vi "Skew_Image2.vi"(4 "[IN] Skewed Image":T1, 5 "[IN] Share Angle":u16 max=89 step=1, 6 "[IN] Calculation mode":enum16{"Single core", "2x cores", "4x cores"}(ring), 7 "error IN":errorcluster, 8 "[IN] Y = Array rows":i32, 9 "[IN] X = Array cols":i32, 10 "[IN] Source Image U16":u16[][](array[numeric])) -> (0 "error OUT":errorcluster, 3 "[OUT] Skewed Image":T1)   [LabVIEW 2020]
uses:
  <vilib>/vision/Image Controls.llb/IMAQ Image.ctl
  <vilib>/vision/NI_Vision_Development_Module.lvlib
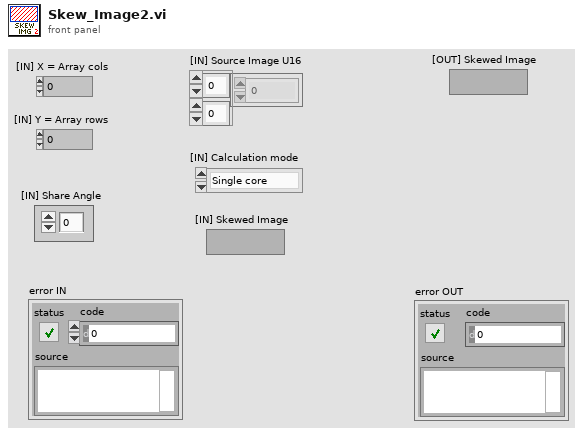
[diagram p1: front panel]
types:
  T1 = typedef "IMAQ Image.ctl" = refnum<image>
  T2 = typedef "Image Type" = u32
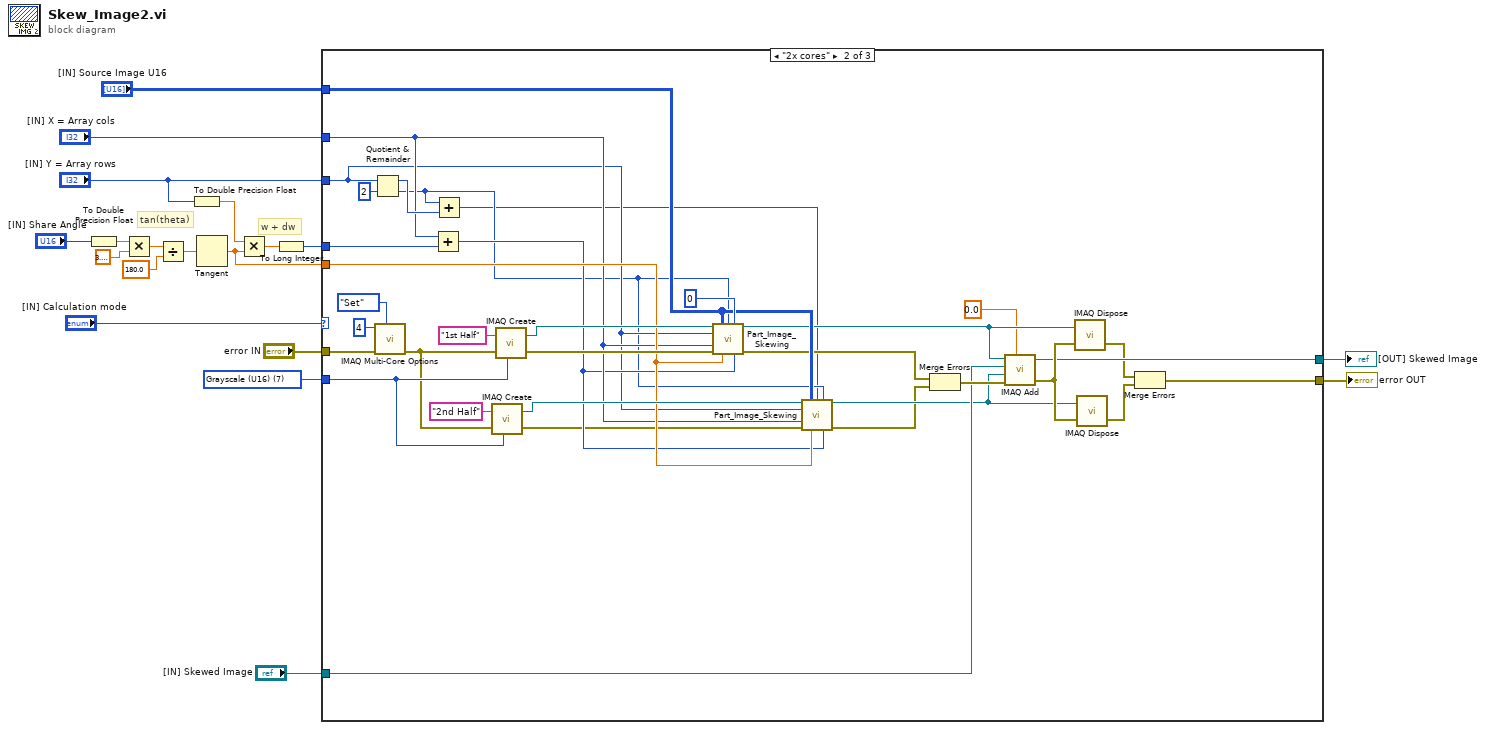
[diagram p0: block diagram]
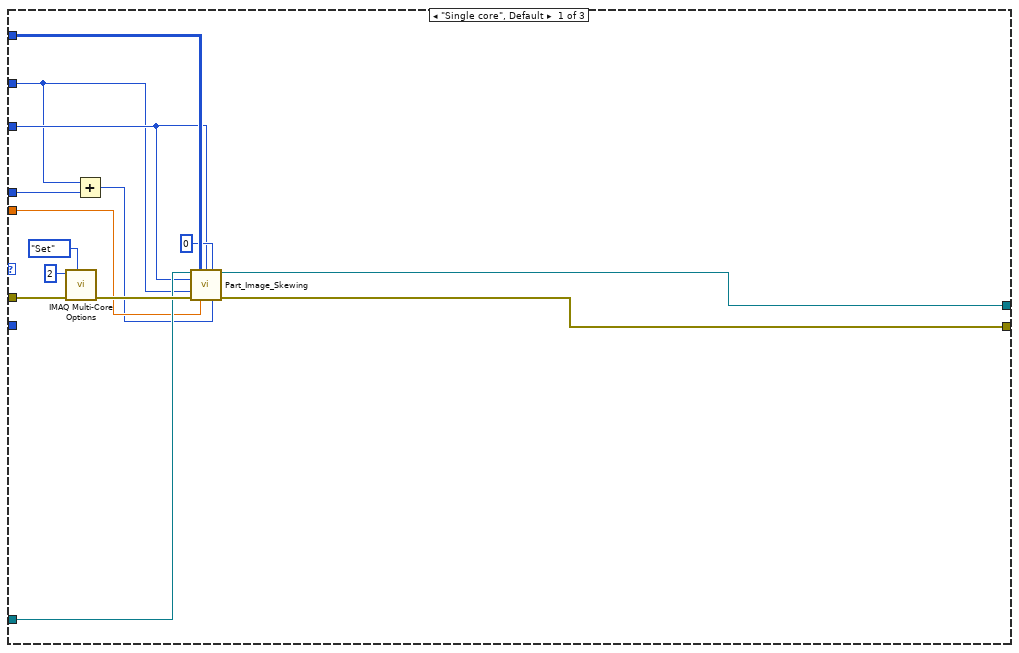
[diagram p2: hidden frame]
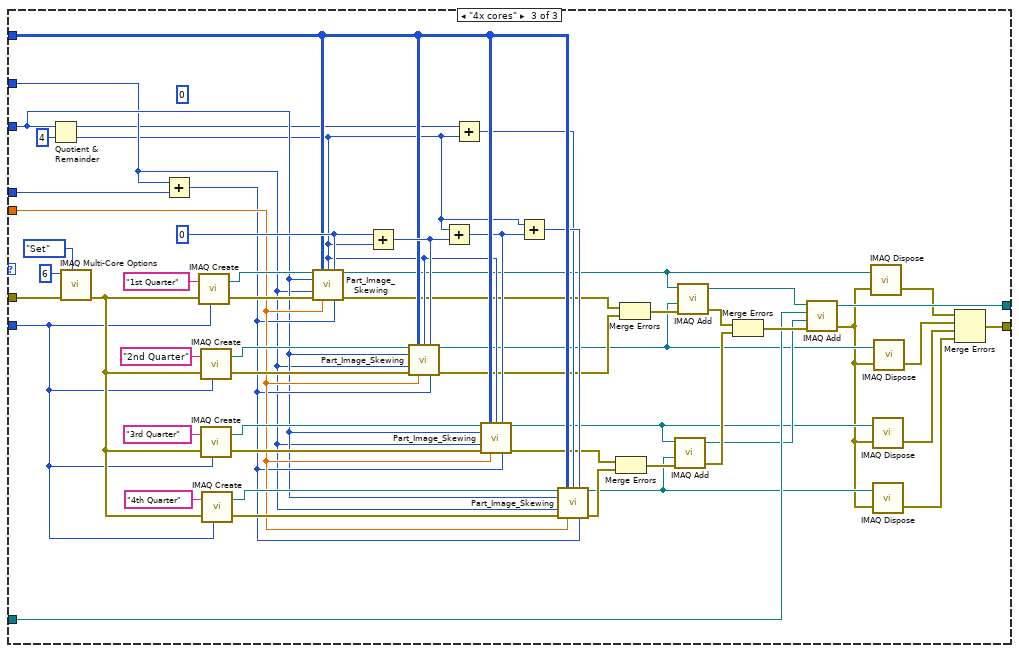
[diagram p3: hidden frame]
diagram:
  w3 = T2 7 items=["Grayscale (U8)", "Grayscale (I16)", "Grayscale (SGL)", "Complex (CSG)", "RGB (U32)", "HSL (U32)", "RGB (U64)", "Grayscale (U16)"] ("Image Type")
  # "w + dw"
  # "tan(theta)"
  n1 = To Double Precision Float(number="[IN] Share Angle") -> (double precision float=w19:dbl)
  n2 = Multiply(x=w19, y=3.141592653589793) -> (x*y=w18:dbl)
  n3 = Divide(x=w18, y=180.0) -> (x/y=w16:dbl)
  n4 = To Double Precision Float(number="[IN] Y = Array rows") -> (double precision float=w10:dbl)
  n5 = Tangent(1:w16) -> (0:w14:dbl)
  n6 = Multiply(x=w10, y=w14) -> (x*y=w13:dbl)
  n7 = To Long Integer(number=w13) -> (32bit integer=w15:i32)
  n8 = case shown="\"2x cores\"" "[IN] Calculation mode" {
    tunnel: w15 -> [w23 w66 w120]
    tunnel: w14 -> [w21 w50 w100]
    tunnel: "[IN] Source Image U16" -> [w28 w53 w96]
    tunnel: "[IN] X = Array cols" -> [w22 w49 w97]
    tunnel: "[IN] Y = Array rows" -> [w24 w39 w98]
    tunnel: "error IN" -> [w31 w59 w117]
    tunnel: [w25 w40 w72] -> w4
    tunnel: w3 -> [_ w60 w111]
    tunnel: [w26 w43 w76] -> w2
    tunnel: "[IN] Skewed Image" -> [w29 w47 w80]
    frame "Single core", Default {
      n9 = call "IMAQ Multi-Core Options"("Get/Set Number of Cores (Get)"=enum32{"Get", "Set", "Set Max Available"}."Set", "error in (no error)"=w31, "Specified Number of Cores"=u32 2) -> ("error out"=w30:errorcluster)  [unwired: 7 in, 1 out]
      n10 = Add(x=w22, y=w23) -> (x+y=w20:i32)
      n11 = call "Part_Image_Skewing.vi"("[IN] Part Image"=w29, "[IN] Source Image U16"=w28, "[IN] Rows Part"=w24, "[IN] Part shift"=0, "[IN] Rows"=w24, "[IN] Cols Initial"=w22, "error IN"=w30, "[IN] tan(theta)"=w21, "[IN] Cols"=w20) -> ("[OUT] Part Image"=w26:T1, "error OUT"=w25:errorcluster)  [unwired: 5 in]
    }
    frame "2x cores" {
      n12 = Quotient & Remainder(x=w39, y=2) -> (x-y*floor(x/y)=w65:i32, floor(x/y)=w37:i32)
      n13 = call "IMAQ Multi-Core Options"("Get/Set Number of Cores (Get)"=enum32{"Get", "Set", "Set Max Available"}."Set", "error in (no error)"=w59, "Specified Number of Cores"=u32 4) -> ("error out"=w58:errorcluster)  [unwired: 7 in, 1 out]
      n14 = Add(x=w49, y=w66) -> (x+y=w48:i32)
      n15 = Add(x=w37, y=w65) -> (x+y=w36:i32)
      n16 = call "IMAQ Create"("Image Name"="2nd Half", "Image Type"=w60, "error in (no error)"=w58) -> ("New Image"=w54:T1, "error out"=w35:errorcluster)  [unwired: 2 in]
      n17 = call "IMAQ Create"("Image Name"="1st Half", "Image Type"=w60, "error in (no error)"=w58) -> ("New Image"=w56:T1, "error out"=w57:errorcluster)  [unwired: 2 in]
      n18 = call "Part_Image_Skewing.vi"("[IN] Part Image"=w56, "[IN] Source Image U16"=w53, "[IN] Rows Part"=w37, "[IN] Part shift"=0, "[IN] Rows"=w39, "[IN] Cols Initial"=w49, "error IN"=w57, "[IN] tan(theta)"=w50, "[IN] Cols"=w48) -> ("[OUT] Part Image"=w46:T1, "error OUT"=w52:errorcluster)  [unwired: 5 in]
      n19 = call "Part_Image_Skewing.vi"("[IN] Part Image"=w54, "[IN] Source Image U16"=w53, "[IN] Rows Part"=w36, "[IN] Part shift"=w37, "[IN] Rows"=w39, "[IN] Cols Initial"=w49, "error IN"=w35, "[IN] tan(theta)"=w50, "[IN] Cols"=w48) -> ("[OUT] Part Image"=w44:T1, "error OUT"=w34:errorcluster)  [unwired: 5 in]
      n20 = Merge Errors(w52, w34) -> (w51:errorcluster)
      n21 = call "IMAQ Add"("Image Src A"=w46, "Constant"=0.0, "Image Dst"=w47, "Image Src B"=w44, "error in (no error)"=w51) -> ("Image Dst Out"=w43:T1, "error out"=w45:errorcluster)  [unwired: 2 in]
      n22 = call "IMAQ Dispose"("Image"=w46, "error in (no error)"=w45) -> ("error out"=w42:errorcluster)  [unwired: 4 in]
      n23 = call "IMAQ Dispose"("Image"=w44, "error in (no error)"=w45) -> ("error out"=w41:errorcluster)  [unwired: 4 in]
      n24 = Merge Errors(w42, w41) -> (w40:errorcluster)
    }
    frame "4x cores" {
      w108 = 0 ("[IN] Part shift")
      (unwired) u16 0
      n25 = Quotient & Remainder(x=w98, y=4) -> (x-y*floor(x/y)=w93:i32, floor(x/y)=w91:i32)
      n26 = call "IMAQ Multi-Core Options"("Get/Set Number of Cores (Get)"=enum32{"Get", "Set", "Set Max Available"}."Set", "error in (no error)"=w117, "Specified Number of Cores"=u32 6) -> ("error out"=w112:errorcluster)  [unwired: 7 in, 1 out]
      n27 = Add(x=w97, y=w120) -> (x+y=w99:i32)
      n28 = call "IMAQ Create"("Image Name"="1st Quarter", "Image Type"=w111, "error in (no error)"=w112) -> ("New Image"=w109:T1, "error out"=w110:errorcluster)  [unwired: 2 in]
      n29 = call "IMAQ Create"("Image Name"="2nd Quarter", "Image Type"=w111, "error in (no error)"=w112) -> ("New Image"=w106:T1, "error out"=w107:errorcluster)  [unwired: 2 in]
      n30 = call "IMAQ Create"("Image Name"="3rd Quarter", "Image Type"=w111, "error in (no error)"=w112) -> ("New Image"=w104:T1, "error out"=w105:errorcluster)  [unwired: 2 in]
      n31 = call "IMAQ Create"("Image Name"="4th Quarter", "Image Type"=w111, "error in (no error)"=w112) -> ("New Image"=w101:T1, "error out"=w102:errorcluster)  [unwired: 2 in]
      n32 = call "Part_Image_Skewing.vi"("[IN] Part Image"=w109, "[IN] Source Image U16"=w96, "[IN] Rows Part"=w91, "[IN] Part shift"=w108, "[IN] Rows"=w98, "[IN] Cols Initial"=w97, "error IN"=w110, "[IN] tan(theta)"=w100, "[IN] Cols"=w99) -> ("[OUT] Part Image"=w78:T1, "error OUT"=w90:errorcluster)  [unwired: 5 in]
      n33 = Add(x=w108, y=w91) -> (x+y=w103:i32)
      n34 = call "Part_Image_Skewing.vi"("[IN] Part Image"=w106, "[IN] Source Image U16"=w96, "[IN] Rows Part"=w91, "[IN] Part shift"=w103, "[IN] Rows"=w98, "[IN] Cols Initial"=w97, "error IN"=w107, "[IN] tan(theta)"=w100, "[IN] Cols"=w99) -> ("[OUT] Part Image"=w77:T1, "error OUT"=w89:errorcluster)  [unwired: 5 in]
      n35 = Add(x=w91, y=w103) -> (x+y=w95:i32)
      n36 = Add(x=w93, y=w91) -> (x+y=w92:i32)
      n37 = call "Part_Image_Skewing.vi"("[IN] Part Image"=w104, "[IN] Source Image U16"=w96, "[IN] Rows Part"=w91, "[IN] Part shift"=w95, "[IN] Rows"=w98, "[IN] Cols Initial"=w97, "error IN"=w105, "[IN] tan(theta)"=w100, "[IN] Cols"=w99) -> ("[OUT] Part Image"=w75:T1, "error OUT"=w87:errorcluster)  [unwired: 5 in]
      n38 = Add(x=w91, y=w95) -> (x+y=w94:i32)
      n39 = call "Part_Image_Skewing.vi"("[IN] Part Image"=w101, "[IN] Source Image U16"=w96, "[IN] Rows Part"=w92, "[IN] Part shift"=w94, "[IN] Rows"=w98, "[IN] Cols Initial"=w97, "error IN"=w102, "[IN] tan(theta)"=w100, "[IN] Cols"=w99) -> ("[OUT] Part Image"=w74:T1, "error OUT"=w86:errorcluster)  [unwired: 5 in]
      n40 = Merge Errors(w87, w86) -> (w85:errorcluster)
      n41 = Merge Errors(w90, w89) -> (w88:errorcluster)
      n42 = call "IMAQ Add"("Image Src A"=w75, "Image Src B"=w74, "error in (no error)"=w85) -> ("Image Dst Out"=w79:T1, "error out"=w83:errorcluster)  [unwired: 4 in]
      n43 = call "IMAQ Add"("Image Src A"=w78, "Image Src B"=w77, "error in (no error)"=w88) -> ("Image Dst Out"=w81:T1, "error out"=w84:errorcluster)  [unwired: 4 in]
      n44 = Merge Errors(w84, w83) -> (w82:errorcluster)
      n45 = call "IMAQ Add"("Image Src A"=w81, "Image Dst"=w80, "Image Src B"=w79, "error in (no error)"=w82) -> ("Image Dst Out"=w76:T1, "error out"=w73:errorcluster)  [unwired: 3 in]
      n46 = call "IMAQ Dispose"("Image"=w78, "error in (no error)"=w73) -> ("error out"=w71:errorcluster)  [unwired: 4 in]
      n47 = call "IMAQ Dispose"("Image"=w75, "error in (no error)"=w73) -> ("error out"=w69:errorcluster)  [unwired: 4 in]
      n48 = call "IMAQ Dispose"("Image"=w74, "error in (no error)"=w73) -> ("error out"=w68:errorcluster)  [unwired: 4 in]
      n49 = call "IMAQ Dispose"("Image"=w77, "error in (no error)"=w73) -> ("error out"=w70:errorcluster)  [unwired: 4 in]
      n50 = Merge Errors(w71, w70, w69, w68) -> (w72:errorcluster)
    }
  }
  "error OUT" <- w4
  "[OUT] Skewed Image" <- w2
